vi "TCPIPCOMUNICATION.vi"() -> ()   [LabVIEW 2020]
panel:
  out "number 2":dbl
  out "Waveform Chart 2":dbl(graph)
  out "number":dbl
  out "Waveform Chart":dbl(graph)
  in  "stop":bool
  in  "address":string
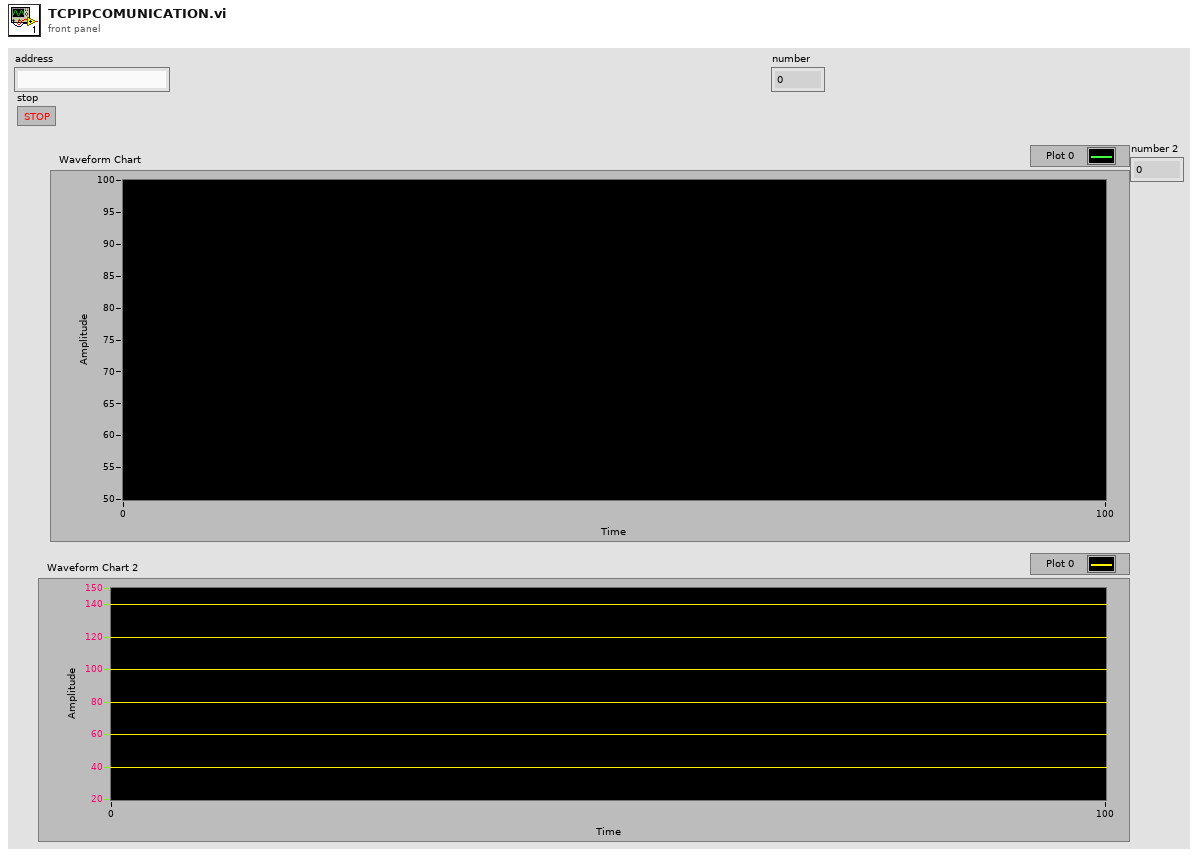
[diagram p1: front panel]
types:
  T1 = enum16{"Standard", "Buffered", "CRLF", "Immediate"}
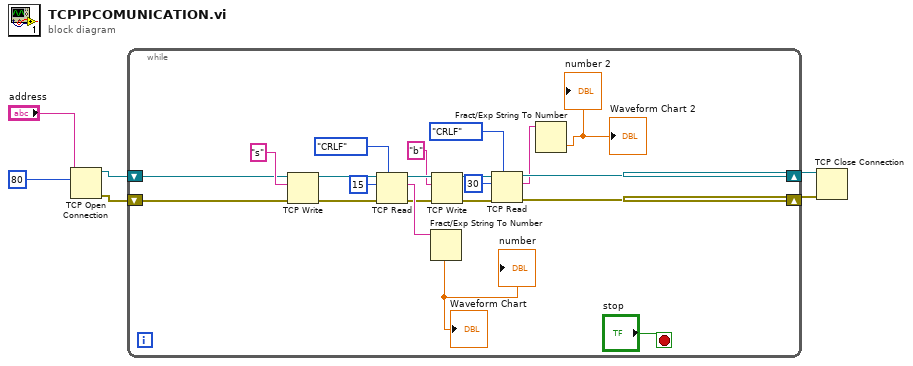
[diagram p0: block diagram]
diagram:
  n1 = TCP Open Connection(address="address", remote port or service name=u16 80) -> (connection ID=w1:refnum<k5>, error out=w2:errorcluster)  [unwired: 3 in]
  n2 = while {
    shift-right: [w9] -> w6
    shift-left: w2 -> [w22]
    shift-right: [w10] -> w5
    shift-left: w1 -> [w21]
    stop <- "stop" stop-if-true
    n3 = TCP Write(connection ID=w21, data in="s", error in (no error)=w22) -> (connection ID out=w27:refnum<k5>, error out=w26:errorcluster)  [unwired: 1 in, 1 out]
    n4 = TCP Read(connection ID=w27, bytes to read=15, error in (no error)=w26, 7:T1."CRLF" ("mode (standard)")) -> (connection ID out=w17:refnum<k5>, data out=w19:string, error out=w16:errorcluster)  [unwired: 1 in]
    n5 = Fract/Exp String To Number(string=w19) -> (number=→"Waveform Chart" →"number":dbl)  [unwired: 3 in, 1 out]
    n6 = TCP Write(connection ID=w17, data in="b", error in (no error)=w16) -> (connection ID out=w15:refnum<k5>, error out=w14:errorcluster)  [unwired: 1 in, 1 out]
    n7 = TCP Read(connection ID=w15, bytes to read=30, error in (no error)=w14, 7:T1."CRLF" ("mode (standard)")) -> (connection ID out=w10:refnum<k5>, data out=w8:string, error out=w9:errorcluster)  [unwired: 1 in]
    n8 = Fract/Exp String To Number(string=w8) -> (number=→"Waveform Chart 2" →"number 2":dbl)  [unwired: 3 in, 1 out]
  }
  n9 = TCP Close Connection(connection ID=w5, error in (no error)=w6) -> ()  [unwired: 1 in, 2 out]
